vi "Botones_intensidad_automatico.vi"(7 "Directorio scripts matlab 2":path=path "C:/Users/franjas/Documents/rutinas-calibracion-slm", 8 "Angulo elementos ópticos":dbl[](array[numeric]), 9 "Nombre de archivo":string, 10 "Seleción método":bool, 11 "Run":bool) -> (5 "?":bool)   [LabVIEW 2013]
uses:
  <vilib>/regexp/Match Regular Expression.xnode
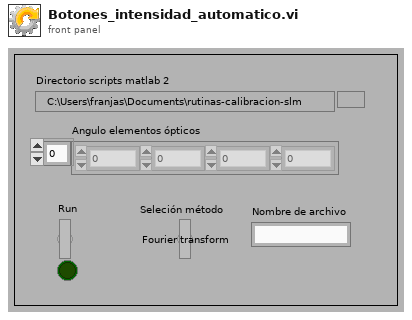
[diagram p1: front panel]
types:
  T1 = enum16{"Escritura", "Med fas F", "Conf fas F", "Med fas IPS", "Conf fas IPS", "Med ampl", "Conf final", "finalizar"}
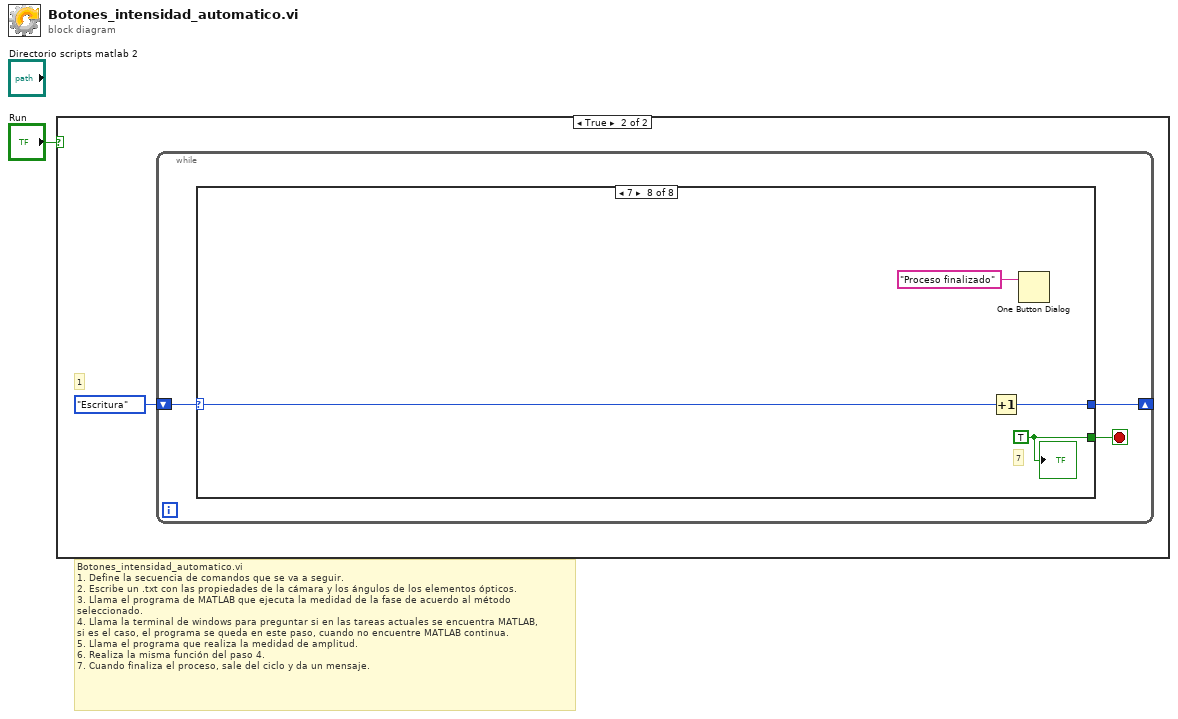
[diagram p0: block diagram]
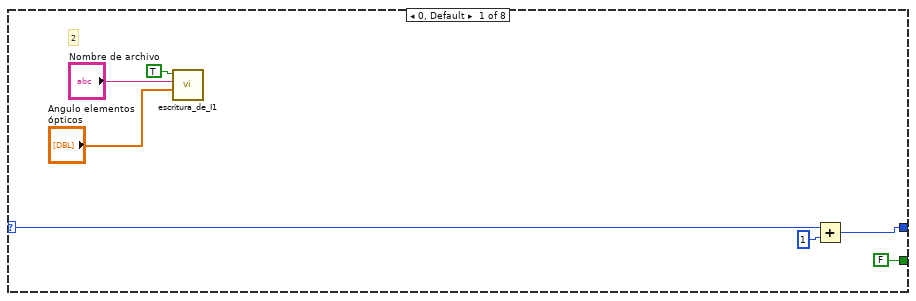
[diagram p3: hidden frame]
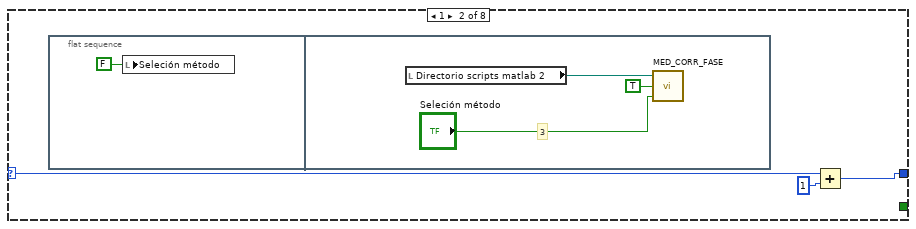
[diagram p4: hidden frame]
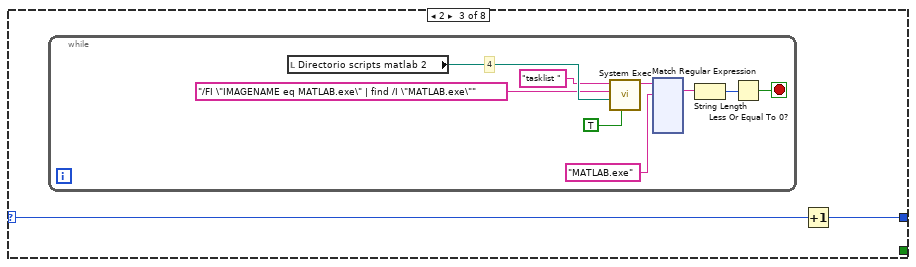
[diagram p5: hidden frame]
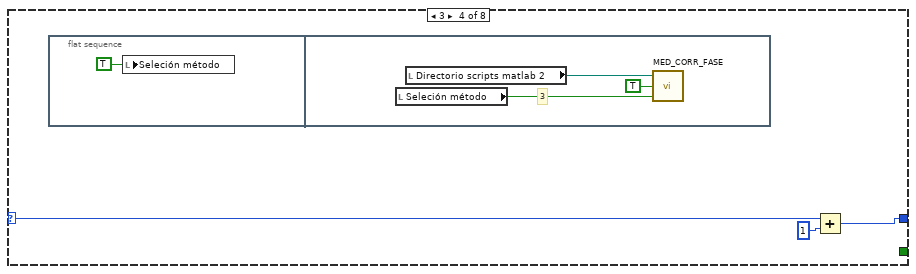
[diagram p6: hidden frame]
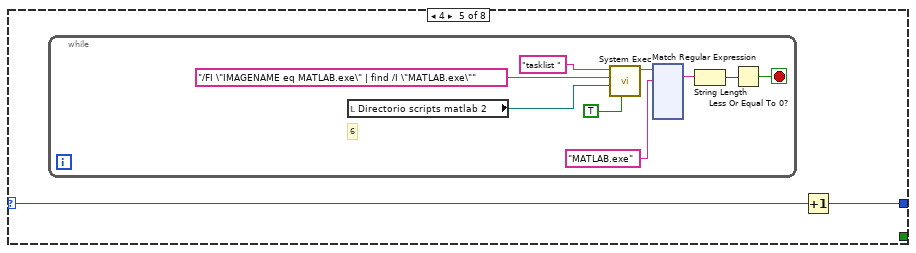
[diagram p7: hidden frame]
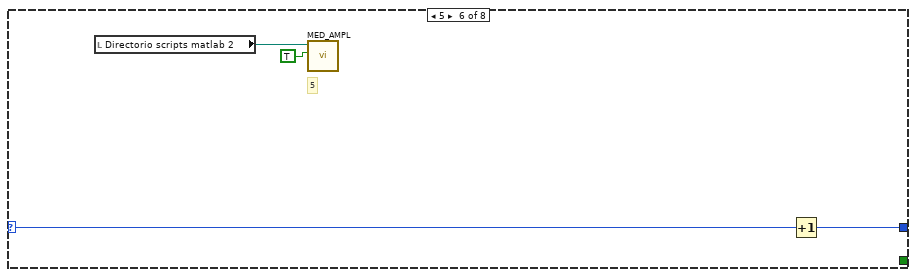
[diagram p8: hidden frame]
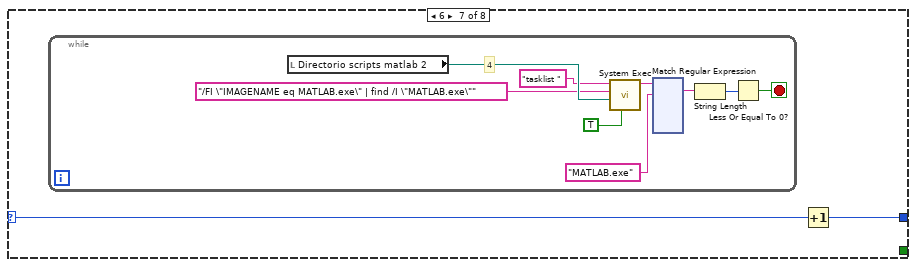
[diagram p9: hidden frame]
diagram:
  # "Botones_intensidad_automatico.vi\n1. Define la secuencia de comandos que se va a seguir.\n2. Escribe un .txt con las propiedades de la cámara y los ángulos de los elementos ópticos.\n3. Llama el programa de MATLAB que ejecuta la medidad de la fase de acuerdo al método \nseleccionado. \n4. Llama la terminal de windows para preguntar si en las tareas actuales se encuentra MATLAB,\nsi es el caso, el programa se queda en este paso, cuando no encuentre MATLAB continua.\n5. Llama el programa que realiza la medidad de amplitud.\n6. Realiza la misma función del paso 4.\n7. Cuando finaliza el proceso, sale del ciclo y da un mensaje."
  n1 = case shown="True" "Run" {
    frame False {
    }
    frame True {
      # "1"
      n2 = while {
        shift-right: [w4] -> _
        shift-left: T1."Escritura" -> [w5]
        stop <- w3 stop-if-true
        n3 = case shown="7" w5 {
          selector: w5 -> [w11 w14 w20 w149 w155 w283 w287 w417]
          tunnel: [w12 w13 w21 w148 w156 w284 w288 w418] -> w4
          tunnel: [FALSE ("I1\n<0,0|0,0>") _ _ _ _ _ _ w416] -> w3
          frame 0, Default {
            # "2"
            n4 = call "escritura_de_I1.vi"("I1\n<0,0|0,0>"=TRUE ("I1\n<0,0|0,0>"), "String"="Nombre de archivo", "Array"="Angulo elementos ópticos") -> ()  [unwired: 8 in]
            n5 = Add(x=w11, y=1) -> (x+y=w12:i32)
          }
          frame 1 {
            n6 = flat-sequence {
              frame #0 {
                n7 = local write "Seleción método"(FALSE ("Seleción método")) -> ()
              }
              frame #1 {
                # "3"
                n8 = local read "Directorio scripts matlab 2"() -> (w17:path)
                n9 = call "MED_CORR_FASE.vi"("Seleción método"="Seleción método", "Ejecucion"=TRUE, "Directorio scripts matlab"=w17) -> ()
              }
            }
            n10 = Add(x=w14, y=1) -> (x+y=w13:i32)
          }
          frame 2 {
            n11 = while {
              stop <- w26 stop-if-true
              # "4"
              n12 = local read "Directorio scripts matlab 2"() -> (w30:path)
              n13 = call <vilib>:"System Exec.vi"("run minimized? (F)"=TRUE, "working directory"=w30, "standard input"="/FI \"IMAGENAME eq MATLAB.exe\" | find /I \"MATLAB.exe\"", "command line"="tasklist ") -> ("standard output"=w29:string)  [unwired: 4 in, 3 out]
              n14 = xnode "Match Regular Expression"("input string"=w29, "regular expression"="MATLAB.exe") -> ("whole match"=w25:string)  [unwired: 4 in, 6 out]
              n15 = String Length(string=w25) -> (length=w27:i32)
              n16 = Less Or Equal To 0?(x=w27) -> (x <= 0?=w26:bool)
            }
            n17 = Increment(x=w20) -> (x+1=w21:i32)
          }
          frame 3 {
            n18 = flat-sequence {
              frame #0 {
                n19 = local write "Seleción método"(TRUE ("Seleción método")) -> ()
              }
              frame #1 {
                # "3"
                n20 = local read "Seleción método"() -> (w154:bool)
                n21 = local read "Directorio scripts matlab 2"() -> (w153:path)
                n22 = call "MED_CORR_FASE.vi"("Seleción método"=w154, "Ejecucion"=TRUE, "Directorio scripts matlab"=w153) -> ()
              }
            }
            n23 = Add(x=w149, y=1) -> (x+y=w148:i32)
          }
          frame 4 {
            n24 = while {
              stop <- w161 stop-if-true
              # "6"
              n25 = local read "Directorio scripts matlab 2"() -> (w165:path)
              n26 = call <vilib>:"System Exec.vi"("run minimized? (F)"=TRUE, "working directory"=w165, "standard input"="/FI \"IMAGENAME eq MATLAB.exe\" | find /I \"MATLAB.exe\"", "command line"="tasklist ") -> ("standard output"=w164:string)  [unwired: 4 in, 3 out]
              n27 = xnode "Match Regular Expression"("input string"=w164, "regular expression"="MATLAB.exe") -> ("whole match"=w160:string)  [unwired: 4 in, 6 out]
              n28 = String Length(string=w160) -> (length=w162:i32)
              n29 = Less Or Equal To 0?(x=w162) -> (x <= 0?=w161:bool)
            }
            n30 = Increment(x=w155) -> (x+1=w156:i32)
          }
          frame 5 {
            # "5"
            n31 = local read "Directorio scripts matlab 2"() -> (w286:path)
            n32 = call "MED_AMPL.vi"("Run"=TRUE ("Boolean"), "Directorio scripts matlab"=w286) -> ()  [unwired: 10 in]
            n33 = Increment(x=w283) -> (x+1=w284:i32)
          }
          frame 6 {
            n34 = while {
              stop <- w293 stop-if-true
              # "4"
              n35 = local read "Directorio scripts matlab 2"() -> (w297:path)
              n36 = call <vilib>:"System Exec.vi"("run minimized? (F)"=TRUE, "working directory"=w297, "standard input"="/FI \"IMAGENAME eq MATLAB.exe\" | find /I \"MATLAB.exe\"", "command line"="tasklist ") -> ("standard output"=w296:string)  [unwired: 4 in, 3 out]
              n37 = xnode "Match Regular Expression"("input string"=w296, "regular expression"="MATLAB.exe") -> ("whole match"=w292:string)  [unwired: 4 in, 6 out]
              n38 = String Length(string=w292) -> (length=w294:i32)
              n39 = Less Or Equal To 0?(x=w294) -> (x <= 0?=w293:bool)
            }
            n40 = Increment(x=w287) -> (x+1=w288:i32)
          }
          frame 7 {
            w416 = TRUE
            # "7"
            n41 = Increment(x=w417) -> (x+1=w418:i32)
            n42 = One Button Dialog(message="Proceso finalizado") -> ()  [unwired: 1 in, 1 out]
            "?" <- w416
          }
        }
      }
    }
  }
